vi "Get AsciiCmd Array.vi"(8 "error in":errorcluster, 11 "CPC in":refnum<class "CPC.lvclass">) -> (0 "error out":errorcluster, 2 "AsciiCmd":string[](array[string]), 3 "CPC out":refnum<class "CPC.lvclass">)   [LabVIEW 2012, in "CPC.lvclass"]
doc: "Retrieves an array of commands that corresponds to the current CPC implementation."
uses:
  CPC.lvclass
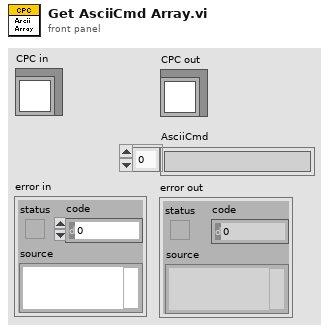
[diagram p1: front panel]
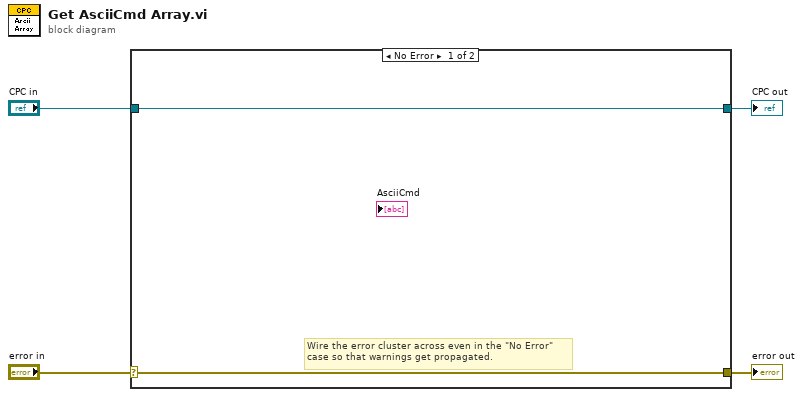
[diagram p0: block diagram]
diagram:
  n1 = case shown="No Error" "error in" {
    selector: "error in" -> [w5 w8]
    tunnel: [w5 w8] -> w3
    tunnel: [w6 w7] -> w1
    tunnel: "CPC in" -> [w6 w7]
    frame No Error {
      # "Wire the error cluster across even in the \"No Error\"\ncase so that warnings get propagated."
    }
    frame Error {
    }
  }
  "error out" <- w3
  "CPC out" <- w1
